vi "GetProperties.vi"(8 "error in":errorcluster, 11 "Enum in":refnum<class "Enum.lvclass">) -> (0 "error out":errorcluster, 3 "Enum out":refnum<class "Enum.lvclass">)   [LabVIEW 2014, in "Enum.lvclass"]
uses:
  Enum.lvclass
  NamedNumeric/NamedNumeric.lvclass
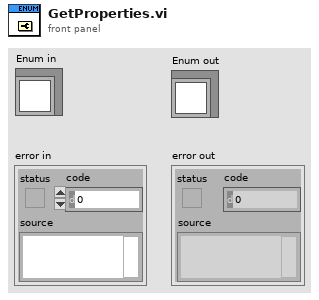
[diagram p1: front panel]
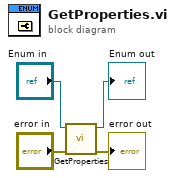
[diagram p0: block diagram]
diagram:
  n1 = call-parent "GetProperties.vi"("error in"="error in", "NamedNumeric in"="Enum in") -> ("error out"=→"error out":errorcluster, "NamedNumeric out"=→"Enum out":refnum<class "Enum.lvclass">)  [unwired: 8 in]
